vi "Find Droplets Freeze Time.vi"(8 "Error In":errorcluster, 10 "GreyLevel Drops and time Derivative in":dbl[][](array[numeric]), 11 "Rel Time Array":u32[](array[numeric])) -> (0 "Error Out":errorcluster, 3 "FreezeYesNo":T1, 4 "DropletBaselineSTD":dbl[](array[numeric]), 6 "DropletBaseline":dbl[](array[numeric]))   [LabVIEW 2013]
uses:
  TypeDef/FreezePointData.ctl
  DB/ConfDB.ctl
  DB/ConfEnum.ctl
  <vilib>/Analysis/NI_AALBase.lvlib
panel:
  out "Derivative":cluster{u32[], "GreyLevelArray":dbl[]}[](graph)
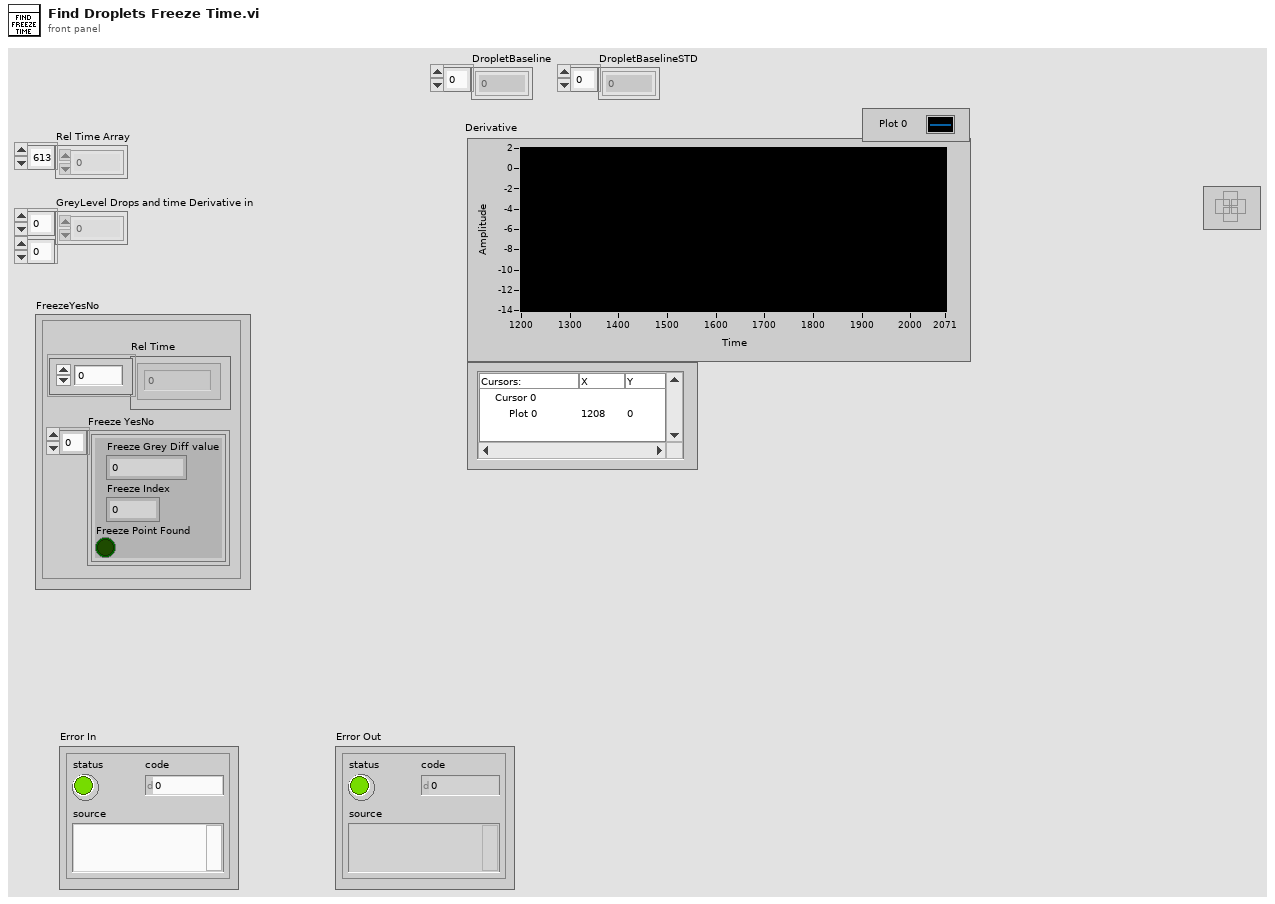
[diagram p1: front panel]
types:
  T1 = typedef "FreezePointData.ctl" = cluster{"Freeze YesNo":cluster{"Freeze Grey Diff value":dbl, "Freeze Index":u32, "Freeze Point Found":bool}[], "Rel Time":u32[]}
  T2 = typedef "ConfEnum.ctl" = enum16{"Init", "GetConfDB", "Configure DB"}
  T3 = typedef "ConfDB.ctl" = cluster{"NumberOfImages":i32, "NoImages2SaveAroundFreeze":i32, "Path":path, "NameOfPartialFile":string, "StartIndex":i32, "NumberOfStdTol":i32, "Detla t (sec)":i32, "Number of images for baseline":i32, "Temperature File Name":string, "Score":dbl, "Index number of Files":i32[], "End Index":i32}
  T4 = cluster{"Minimum value":dbl, "Min Index":u32, "Min Found":bool}[]
  T5 = cluster{"Minimum value":dbl, "Min Index":u32, "Min Found":bool}
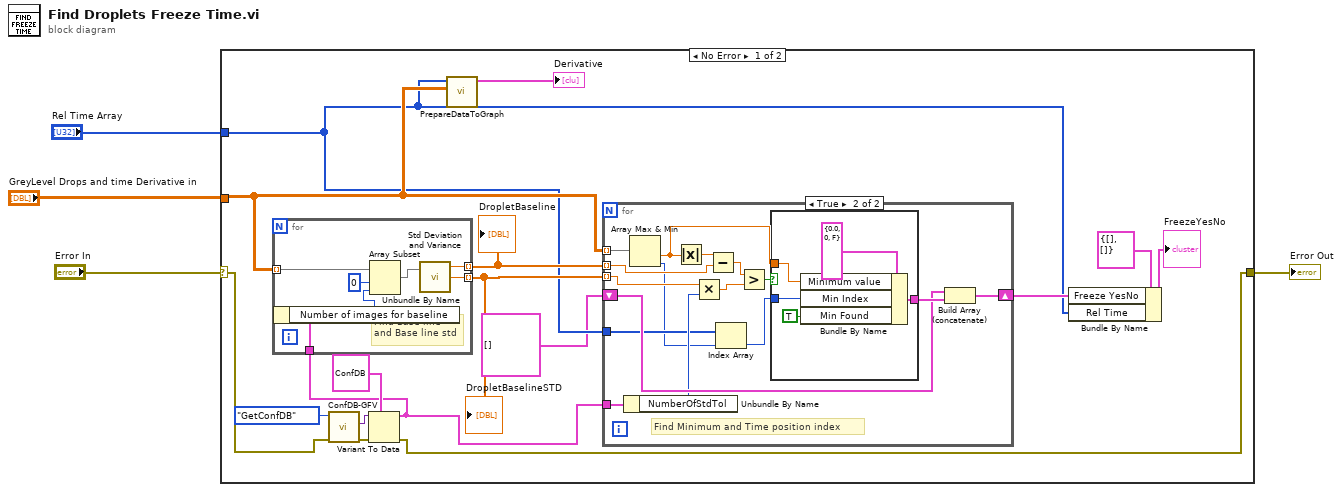
[diagram p0: block diagram]
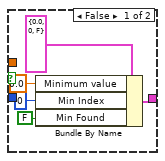
[diagram p2: hidden frame]
diagram:
  n1 = case shown="No Error" "Error In" {
    selector: "Error In" -> [w9 w54]
    tunnel: "Rel Time Array" -> [w6 _]
    tunnel: "GreyLevel Drops and time Derivative in" -> [w18 _]
    tunnel: [w8 w54] -> w1
    frame No Error {
      n2 = call "ConfDB-GFV.vi"("error in (no error)"=w9, "Command In"=ConfEnum."GetConfDB") -> ("error out"=w11:errorcluster, "Data out"=w12:variant)  [unwired: 8 in]
      n3 = Variant To Data(error in=w11, type=T3 {"NumberOfImages"=0, "NoImages2SaveAroundFreeze"=0, "Path"=path "", "NameOfPartialFile"="", "StartIndex"=0, "NumberOfStdTol"=0, "Detla t (sec)"=2, "Number of images for baseline"=0, "Temperature File Name"="", "Score"=0.0, "Index number of Files"=[], "End Index"=0} ("ConfDB"), Variant=w12) -> (data=w7:T3, error out=w8:errorcluster)
      n4 = for {
        tunnel: w18 -> [w47] mode=indexing
        tunnel: [w53] -> w20 mode=indexing
        tunnel: [w52] -> w19 mode=indexing
        tunnel: w7 -> [w50]
        # "Find Base line\nand Base line std"
        n5 = Unbundle By Name(w50) -> ("Number of images for baseline"=w49:i32)
        n6 = Array Subset(array=w47, index=0, length=w49) -> (w51:dbl[])
        n7 = call <vilib>:"Std Deviation and Variance.vi"("X"=w51) -> ("mean"=w53:dbl, "standard deviation"=w52:dbl)  [unwired: 1 in, 1 out]
      }
      "DropletBaseline" <- w20
      "DropletBaselineSTD" <- w19
      n8 = call "PrepareDataToGraph.vi"("GreyLevel Drops and time"=w18, "Rel Time (s)"=w6) -> ("Graph XY data"=→"Derivative":cluster{u32[], "GreyLevelArray":dbl[]}[])  [unwired: 8 in, 1 out]
      n9 = for {
        tunnel: w20 -> [w34] mode=indexing
        tunnel: w19 -> [w32] mode=indexing
        tunnel: w18 -> [w36] mode=indexing
        shift-right: [w28] -> w14
        shift-left: T4 [] -> [w27]
        tunnel: w7 -> [w25]
        tunnel: w6 -> [w23]
        # "Find Minimum and Time position index"
        n10 = Unbundle By Name(w25) -> ("NumberOfStdTol"=w24:i32)
        n11 = Array Max & Min(array=w36) -> (min value=w30:dbl, min index (indices)=w21:i32)  [unwired: 2 out]
        n12 = Absolute Value(x=w30) -> (abs(x)=w35:dbl)
        n13 = Multiply(x=w32, y=w24) -> (x*y=w26:dbl)
        n14 = Subtract(x=w35, y=w34) -> (x-y=w33:dbl)
        n15 = Index Array(array=w23, index=w21) -> (element=w22:u32)
        n16 = Greater?(x=w33, y=w26) -> (0:w31:bool)
        n17 = case shown="True" w31 {
          tunnel: w22 -> [_ w46]
          tunnel: w30 -> [_ w44]
          tunnel: [w39 w43] -> w29
          frame False {
            n18 = Bundle By Name(cluster=T5 {"Minimum value"=0.0, "Min Index"=0, "Min Found"=FALSE} ("Min"), "Minimum value"=0.0, "Min Index"=u32 0, "Min Found"=FALSE) -> (w39:T5)
          }
          frame True {
            n19 = Bundle By Name(cluster=T5 {"Minimum value"=0.0, "Min Index"=0, "Min Found"=FALSE} ("Min"), "Minimum value"=w44, "Min Index"=w46, "Min Found"=TRUE) -> (w43:T5)
          }
        }
        n20 = Build Array (concatenate)(w27, w29) -> (w28:T4)
      }
      n21 = Bundle By Name(cluster=T1 {"Freeze YesNo"=[], "Rel Time"=[]} ("FreezeYesNo"), "Freeze YesNo"=w14, "Rel Time"=w6) -> (→"FreezeYesNo":T1)
    }
    frame Error {
    }
  }
  "Error Out" <- w1
